vi "Configure Horizontal.vi"(8 "error in":errorcluster, 11 "HDO4000A Base CFG in":refnum<class "HDO4000A Base CFG.lvclass">) -> (0 "error out":errorcluster, 3 "HDO4000A Base CFG out":refnum<class "HDO4000A Base CFG.lvclass">)   [LabVIEW 2023, in "HDO4000A Base CFG.lvclass"]
uses:
  HDO4000A Base CFG.lvclass
  D:/git/HAL/Configuration Base/Configuration Base.lvclass
  D:/git/HAL/Scope VISA/Configuration/Scope VISA CFG.lvclass
  HAL/Scope VISA/Configuration/Scope VISA CFG.lvclass/Scope VISA CFG.ctl
  HAL/Configuration Base/Configuration Base.lvclass/Configuration Base.ctl
  18b79182-60ac-4337-870c-577d9c385722.vi
  7a370620-5535-4ad9-8bae-86593e017d87.vi
  50f99c01-86d6-48b7-8ad1-9f25e6893f96.vi
  4f2ba79a-86ec-45a9-aa6c-6feaf85bcb12.vi
  <vilib>/JDP Science/JSONtext/Find Item.vi
  <vilib>/JDP Science/JSONtext/Next JSON Value.vi
  <vilib>/JDP Science/JSONtext/String Subset.vi
  <vilib>/JDP Science/JSONtext/Parsing/Advance past next JSON Value (inlined COPY).vi
  <vilib>/JDP Science/JSONtext/Parsing/Advance past whitespace.vi
  <vilib>/JDP Science/JSONtext/Parsing/Advance past String.vi
  <vilib>/JDP Science/JSONtext/Parsing/Advance past Number.vi
  <vilib>/JDP Science/JSONtext/Parsing/Advance past Line Ending.vi
  <vilib>/JDP Science/JSONtext/Parsing/Parse Full Path or Item Name.vi
  <vilib>/JDP Science/JSONtext/Parsing/Advance past Array.vi
  <vilib>/JDP Science/JSONtext/Parsing/Advance past Object.vi
  <vilib>/JDP Science/JSONtext/support/Error Cluster From Code.vi
  <vilib>/JDP Science/JSONtext/Offset/Find Item Locations by Path.vi
  <vilib>/JDP Science/JSONtext/JSON text to Variant.vi
  <vilib>/Utility/error.llb/Error Cluster From Error Code.vi
  <vilib>/JDP Science/JSONtext/LVClass Serializer/JSONtext LVClass Serializer.lvclass
  <vilib>/ErrorRing/Error Ring.xnode
  HDO4000A Base CFG.lvclass/HDO4000A Base CFG.ctl
  <instrlib>/LeCroy Wave Series/LeCroy Wave Series.lvlib
  HAL/Configuration Base/Configuration Base.lvclass
  HAL/Scope VISA/Configuration/Scope VISA CFG.lvclass
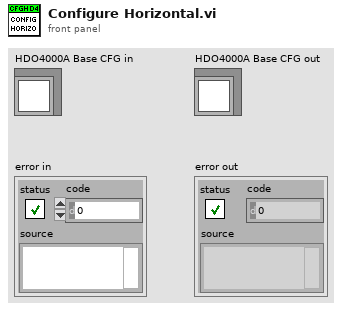
[diagram p1: front panel]
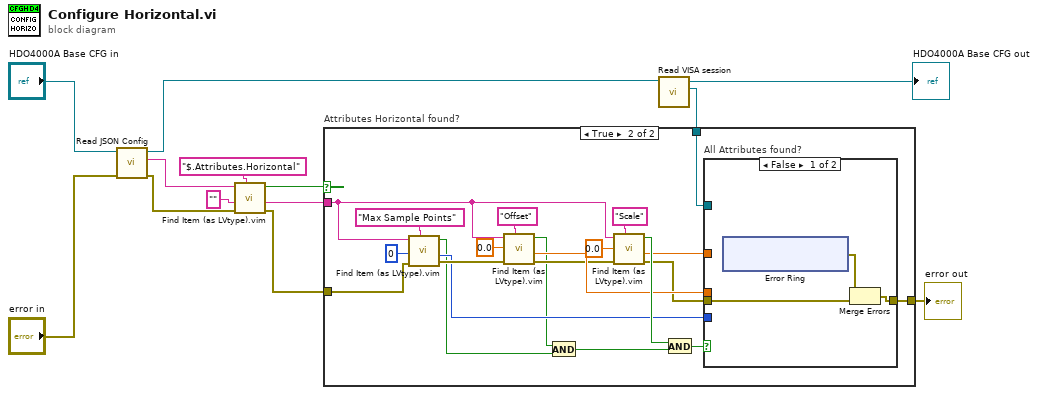
[diagram p0: block diagram]
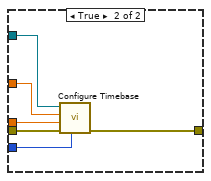
[diagram p3: hidden frame]
diagram:
  n1 = call "Read JSON Config.vi"("error in (no error)"="error in", "object in"="HDO4000A Base CFG in") -> ("error out"=w10:errorcluster, "<JSON>Config"=w9:string, "object out"=w3:refnum<class "HDO4000A Base CFG.lvclass">)  [unwired: 7 in]
  n2 = call "Find Item (as LVtype).vim"("$Path or Item Name"="$.Attributes.Horizontal", "error in (no error)"=w10, "Data Type and Default Value"="", "JSON"=w9) -> ("error out"=w6:errorcluster, "Data"=w7:string, "Found"=w8:bool)  [unwired: 4 in, 1 out]
  n3 = call "Read VISA session.vi"("Scope VISA CFG in"=w3) -> ("VISA session"=w2:refnum<visa-resource-name>, "Scope VISA CFG out"=→"HDO4000A Base CFG out":refnum<class "HDO4000A Base CFG.lvclass">)  [unwired: 8 in, 1 out]
  n4 = case "Attributes Horizontal found?" shown="True" w8 {
    tunnel: w7 -> [_ w23]
    tunnel: w6 -> [w14 w22]
    tunnel: w2 -> [_ w29]
    tunnel: [w14 w15] -> w1
    frame False {
    }
    frame True {
      n5 = call "Find Item (as LVtype).vim"("$Path or Item Name"="Max Sample Points", "error in (no error)"=w22, "Data Type and Default Value"=0, "JSON"=w23) -> ("error out"=w21:errorcluster, "Data"=w19:i32, "Found"=w18:bool)  [unwired: 4 in, 1 out]
      n6 = call "Find Item (as LVtype).vim"("$Path or Item Name"="Offset", "error in (no error)"=w21, "Data Type and Default Value"=0.0, "JSON"=w23) -> ("error out"=w20:errorcluster, "Data"=w28:dbl, "Found"=w17:bool)  [unwired: 4 in, 1 out]
      n7 = And(x=w17, y=w18) -> (x .and. y?=w16:bool)
      n8 = call "Find Item (as LVtype).vim"("$Path or Item Name"="Scale", "error in (no error)"=w20, "Data Type and Default Value"=0.0, "JSON"=w23) -> ("error out"=w26:errorcluster, "Data"=w27:dbl, "Found"=w31:bool)  [unwired: 4 in, 1 out]
      n9 = And(x=w31, y=w16) -> (x .and. y?=w30:bool)
      n10 = case "All Attributes found?" shown="False" w30 {
        tunnel: w29 -> [_ w49]
        tunnel: w28 -> [_ w46]
        tunnel: w27 -> [_ w47]
        tunnel: w26 -> [w37 w48]
        tunnel: w19 -> [_ w45]
        tunnel: [w36 w44] -> w15
        frame False {
          n11 = xnode "Error Ring"() -> ("error out"=w38:errorcluster)
          n12 = Merge Errors(w38, w37) -> (w36:errorcluster)
        }
        frame True {
          n13 = call <instrlib>:"Configure Timebase.vi"("Maximum Sample Points (500)"=w45, "error in (no error)"=w48, "Position (0.0 s)"=w46, "Timebase (0.0005 s)"=w47, "VISA resource name"=w49) -> ("error out"=w44:errorcluster)  [unwired: 5 in, 1 out]
        }
      }
    }
  }
  "error out" <- w1
